vi "Test Array Datatype.vi"(8 "error in (no error)":errorcluster) -> (0 "error out":errorcluster)   [LabVIEW 2018, in "JSON to LVConstant Test.lvlib"]
uses:
  JSON to LVConstant Test.lvlib
  <vilib>/addons/_JKI Toolkits/Caraya/classes/Test/Test.lvclass
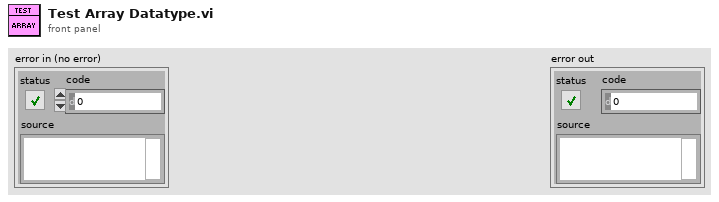
[diagram p1: front panel]
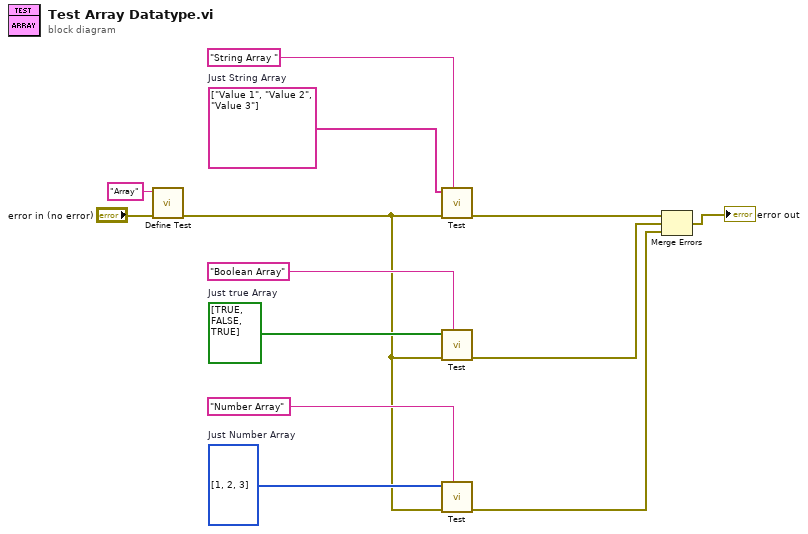
[diagram p0: block diagram]
diagram:
  w4 = i32[] [1, 2, 3]  # Just Number Array
  w6 = bool[] [TRUE, FALSE, TRUE]  # Just true Array
  w12 = string[] ["Value 1", "Value 2", "Value 3"]  # Just String Array
  n1 = call <vilib>:"Define Test.vi"("error in (no error)"="error in (no error)", "Label (VI Title)"="Array") -> ("error out"=w2:errorcluster)  [unwired: 9 in]
  n2 = call "Test.vi"("Label (VI Title)"="String Array ", "error in (no error)"=w2, "Type"=w12) -> ("error out"=w10:errorcluster)  [unwired: 8 in]
  n3 = call "Test.vi"("Label (VI Title)"="Boolean Array", "error in (no error)"=w2, "Type"=w6) -> ("error out"=w7:errorcluster)  [unwired: 8 in]
  n4 = call "Test.vi"("Label (VI Title)"="Number Array", "error in (no error)"=w2, "Type"=w4) -> ("error out"=w5:errorcluster)  [unwired: 8 in]
  n5 = Merge Errors(w10, w7, w5) -> (→"error out":errorcluster)
